vi "PicoScope-3000 Read.vi"(2 "WFD-Ref Ch-B":refnum<vi>, 3 "WFD-Ref Ch-A":refnum<vi>, 4 "Acquisition Settings":T4={"preTriggerSamples"=0, "postTriggerSamples"=10000, "timebase"=5000, "Down-Sample Mode"=0, "Down Sample Ratio"=1} {"Down Sample Ratio" min=1 step=1; "Down-Sample Mode" items=["None"=0, "Aggregate"=1, "Decimate"=2, "Average"=4]; "postTriggerSamples" max=10000 step=100}, 5 "Trigger Settings":T5={"Trigger Enabled"=TRUE, "Trigger Source"=enum."Channel A", "Trigger Threshold (Volts)"=0.0, "Trigger Direction"=2, "Trigger Delay (samples)"=0, "Auto Trigger Time (ms)"=1000} {"Trigger Direction" items=["Rising"=2, "Falling"=3]}, 6 "Channel B Settings":T2={"Enabled"=TRUE, "Coupling"=1, "Range"=8, "Analogue Offset"=0.0} {"Range" items=["20 mV"=1, "50 mV"=2, "100 mV"=3, "200 mV"=4, "500 mV"=5, "1 V"=6, "2 V"=7, "5 V"=8, "10 V"=9, "20 V"=10]; "Coupling" items=["AC", "DC"]}, 7 "Channel A Settings":T2={"Enabled"=TRUE, "Coupling"=1, "Range"=7, "Analogue Offset"=0.0} {"Range" items=["20 mV"=1, "50 mV"=2, "100 mV"=3, "200 mV"=4, "500 mV"=5, "1 V"=6, "2 V"=7, "5 V"=8, "10 V"=9, "20 V"=10]; "Coupling" items=["AC", "DC"]}, 8 "error in":errorcluster, 9 "Max Adc value":i16, 10 "Device Info":T1, 11 "handle":i16) -> (0 "error out":errorcluster, 1 "handle":i16)   [LabVIEW 2018]
panel:
  out "Channel B":cluster{i32, "Sample Internal":sgl, dbl[]}(graph)
  out "Properties Panel":T3 {"Max Total Capture Time Available (sec)" format="%.3p"; "Sample Frequency" format="%.3p"; "Sample Internal" format="%.3p"; "Max Samples Available" format="%.3p"; "Total Capture Time (sec)" format="%.3p"}
  out "Channel A":cluster{i32, "Sample Internal":sgl, dbl[]}(graph)
  # "127"
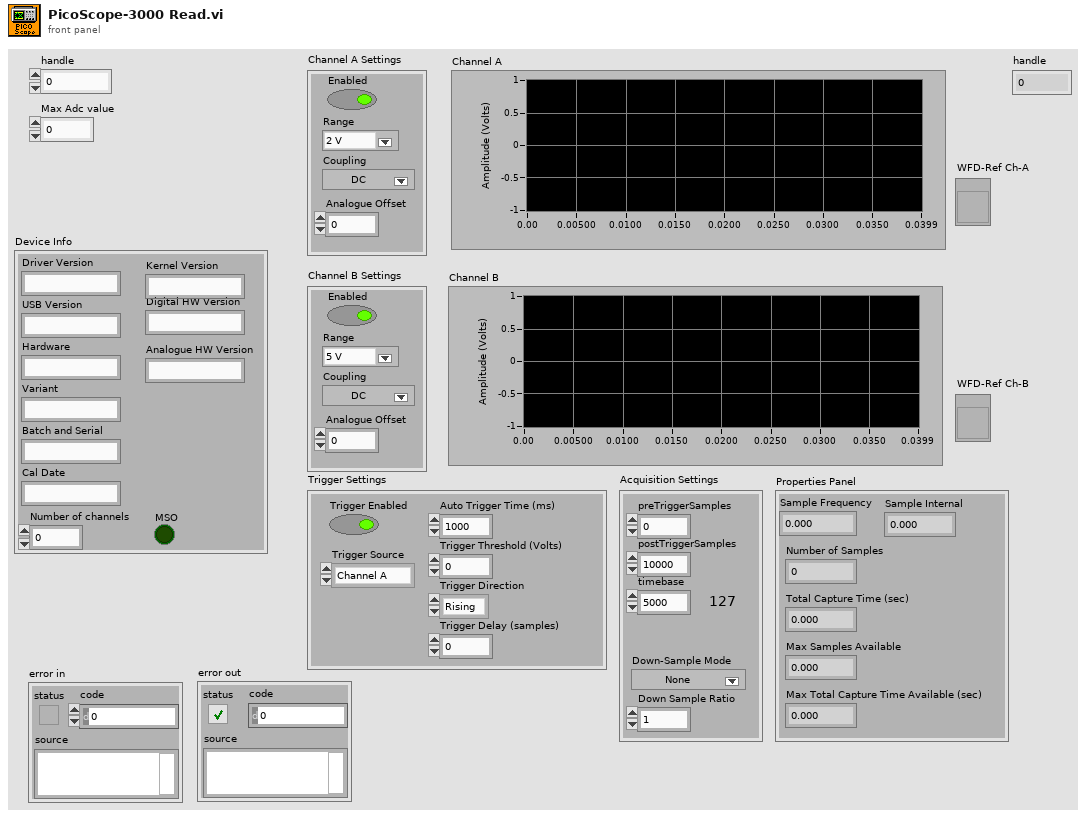
[diagram p1: front panel]
types:
  T1 = cluster{"Driver Version":string, "USB Version":string, "Hardware":string, "Variant":string, "Batch and Serial":string, "Cal Date":string, "Kernel Version":string, "Digital HW Version":string, "Analogue HW Version":string, "MSO":bool, "Number of channels":i16}
  T2 = cluster{"Enabled":bool, "Coupling":i16, "Range":u16, "Analogue Offset":sgl}
  T3 = cluster{"Sample Frequency":sgl, "Sample Internal":sgl, "Max Samples Available":i32, "Number of Samples":u32, "Total Capture Time (sec) ":sgl, "Max Total Capture Time Available (sec)":sgl}
  T4 = cluster{"preTriggerSamples":u32, "postTriggerSamples":u32, "timebase":u32, "Down-Sample Mode":i32, "Down Sample Ratio":u32}
  T5 = cluster{"Trigger Enabled":bool, "Trigger Source":enum16{"Channel A", "Channel B", "Channel C", "Channel D", "Ext."}, "Trigger Threshold (Volts)":dbl, "Trigger Direction":u16, "Trigger Delay (samples)":u32, "Auto Trigger Time (ms)":i16}
  T6 = cluster{"Sample Frequency":sgl, "Sample Rate":sgl, "Max Samples Available":i32, "Number of Samples":u32, "Total Capture Time (sec) ":sgl, "Max Total Capture Time Available (sec)":sgl}
  T7 = cluster{"Channel D Buffer":i16[], "Channel C Buffer":i16[], "Channel B Buffer":i16[], "Channel A Buffer":i16[], "Port 0  Buffer ":i16[], "Port 1 Buffer ":i16[]}
  T8 = cluster{i32, "Sample Rate":sgl, "Data (Volts)":dbl[]}
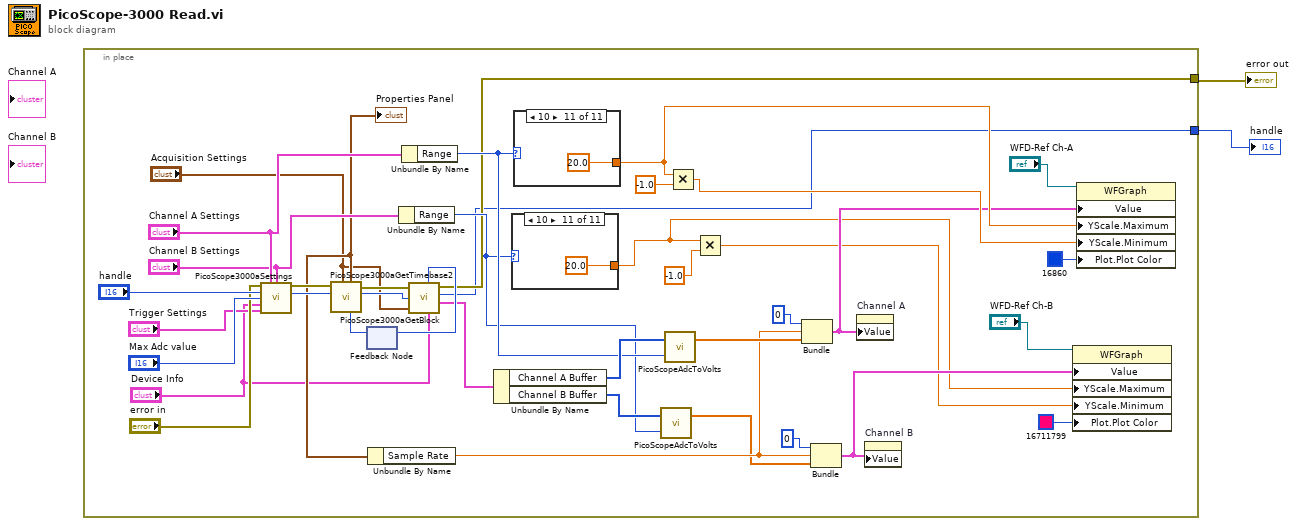
[diagram p0: block diagram]
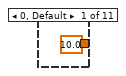
[diagram p2: hidden frame]
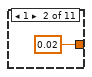
[diagram p3: hidden frame]
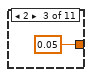
[diagram p4: hidden frame]
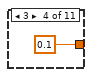
[diagram p5: hidden frame]
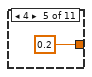
[diagram p6: hidden frame]
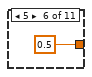
[diagram p7: hidden frame]
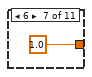
[diagram p8: hidden frame]
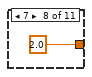
[diagram p9: hidden frame]
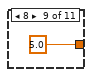
[diagram p10: hidden frame]
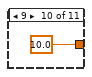
[diagram p11: hidden frame]
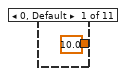
[diagram p12: hidden frame]
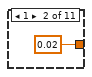
[diagram p13: hidden frame]
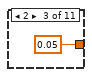
[diagram p14: hidden frame]
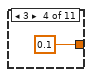
[diagram p15: hidden frame]
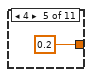
[diagram p16: hidden frame]
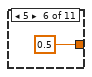
[diagram p17: hidden frame]
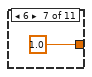
[diagram p18: hidden frame]
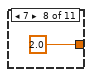
[diagram p19: hidden frame]
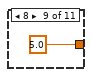
[diagram p20: hidden frame]
diagram:
  n1 = in-place {
    in-place-border: [w9] -> w2
    in-place-border: [w7] -> w1
    n2 = call "PicoScope3000aSettings.vi"("error in"="error in", "Channel A Settings"="Channel A Settings", "Channel B Settings"="Channel B Settings", "handle in"="handle", "Max_adc"="Max Adc value", "Device Info"="Device Info", "Trigger Settings"="Trigger Settings") -> ("error out"=w16:errorcluster, "handle out"=w15:i16)  [unwired: 6 in, 1 out]
    n3 = feedback #1() -> (w14:u32)  [unwired: 1 in]
    n4 = call "PicoScope3000aGetTimebase2.vi"("Number of Samples"=w14, "Acquisition Settings"="Acquisition Settings", "handle in"=w15, "error in (no error)"=w16) -> ("handle out"=w11:i16, "error out"=w12:errorcluster, "Properties Panel"=w13:T6)  [unwired: 5 in]
    "Properties Panel" <- w13
    n5 = Unbundle By Name(w13) -> ("Sample Rate"=w34:sgl)
    n6 = Unbundle By Name("Channel B Settings") -> ("Range"=w26:u16)
    n7 = Unbundle By Name("Channel A Settings") -> ("Range"=w36:u16)
    n8 = call "PicoScope3000aGetBlock.vi"("error in"=w12, "handle in"=w11, "Acquisition Settings"="Acquisition Settings", "Device Info"="Device Info") -> ("noOfSamples"=w10:u32, "error out"=w9:errorcluster, "handle out"=w7:i16, "Buffers (Max or non-aggregated)"=w8:T7)  [unwired: 1 in, 2 out]
    n9 = feedback-in #1(w10) -> ()
    n10 = Unbundle By Name(w8) -> ("Channel A Buffer"=w40:i16[], "Channel B Buffer"=w37:i16[])
    n11 = case shown="10" w26 {
      tunnel: [10.0 0.02 0.05 0.1 0.2 0.5 1.0 2.0 5.0 10.0 20.0] -> w24
      frame 0, Default {
      }
      frame 1 {
      }
      frame 2 {
      }
      frame 3 {
      }
      frame 4 {
      }
      frame 5 {
      }
      frame 6 {
      }
      frame 7 {
      }
      frame 8 {
      }
      frame 9 {
      }
      frame 10 {
      }
    }
    n12 = case shown="10" w36 {
      tunnel: [10.0 0.02 0.05 0.1 0.2 0.5 1.0 2.0 5.0 10.0 20.0] -> w31
      frame 0, Default {
      }
      frame 1 {
      }
      frame 2 {
      }
      frame 3 {
      }
      frame 4 {
      }
      frame 5 {
      }
      frame 6 {
      }
      frame 7 {
      }
      frame 8 {
      }
      frame 9 {
      }
      frame 10 {
      }
    }
    n13 = call "PicoScopeAdcToVolts.vi"("Range Index"=w26, "Data"=w37) -> ("Data (Volts)"=w33:dbl[])  [unwired: 1 in]
    n14 = call "PicoScopeAdcToVolts.vi"("Range Index"=w36, "Data"=w40) -> ("Data (Volts)"=w39:dbl[])  [unwired: 1 in]
    n15 = Multiply(x=w31, y=-1.0) -> (x*y=w30:dbl)
    n16 = Multiply(x=w24, y=-1.0) -> (x*y=w23:dbl)
    n17 = Bundle(0, "Sample Rate"=w34, "Data (Volts)"=w39) -> (w29:T8)  [unwired: 1 in]
    n18 = Bundle(0, "Sample Rate"=w34, "Data (Volts)"=w33) -> (w32:T8)  [unwired: 1 in]
    n19 = property on="Channel A" class="WFGraph (strict)"("Value"=w29) -> ()  [unwired: 2 in, 2 out]
    n20 = property on="Channel B" class="WFGraph (strict)"("Value"=w32) -> ()  [unwired: 2 in, 2 out]
    n21 = property class="WFGraph"(reference="WFD-Ref Ch-B", "Value"=w32, "YScale.Maximum"=w24, "YScale.Minimum"=w23, "Plot.Plot Color"=u32 16711799) -> ()  [unwired: 1 in, 2 out]
    n22 = property class="WFGraph"(reference="WFD-Ref Ch-A", "Value"=w29, "YScale.Maximum"=w31, "YScale.Minimum"=w30, "Plot.Plot Color"=u32 16860) -> ()  [unwired: 1 in, 2 out]
  }
  "error out" <- w2
  "handle" <- w1
